vi "Set Server State UE.vi"(10 "Server State UE":refnum<user-event>, 11 "Template Server in":refnum<class "ctet_dio.lvclass">) -> (3 "Template Server out":refnum<class "ctet_dio.lvclass">)   [LabVIEW 2019, in "ctet_dio.lvlib" / "ctet_dio.lvclass"]
uses:
  ctet_dio.lvclass
  typeDefs/Server State Data.ctl
  ctet_dio.lvclass/ctet_dio.ctl
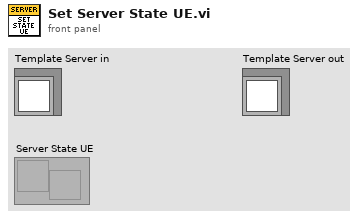
[diagram p1: front panel]
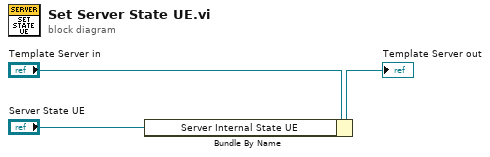
[diagram p0: block diagram]
diagram:
  n1 = Bundle By Name(cluster="Template Server in", "Server Internal State UE"="Server State UE") -> (→"Template Server out":refnum<class "ctet_dio.lvclass">)
